vi "Write Credentials.vi"(8 "error in (no error)":errorcluster, 10 "Credentials":T1, 11 "AWS Core in":refnum<class "AWS Core.lvclass">) -> (0 "error out":errorcluster, 3 "AWS Core out":refnum<class "AWS Core.lvclass">)   [LabVIEW 2015, in "AWS Core.lvlib" / "AWS Core.lvclass"]
uses:
  AWS Core.lvclass
  AWS Credentials.ctl
  AWS Core.lvclass/AWS Core.ctl
  AWS Core.lvlib
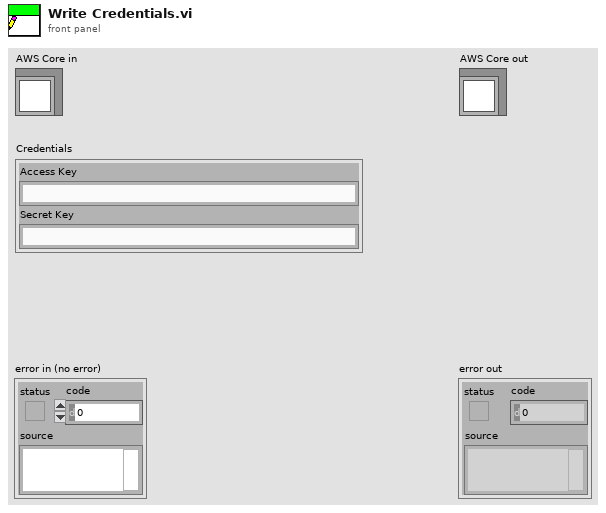
[diagram p1: front panel]
types:
  T1 = typedef "AWS Core.lvlib/AWS Credentials.ctl" = cluster{"Access Key":string, "Secret Key":string}
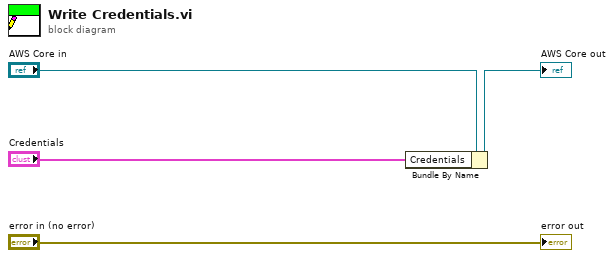
[diagram p0: block diagram]
diagram:
  n1 = Bundle By Name(cluster="AWS Core in", "Credentials"="Credentials") -> (→"AWS Core out":refnum<class "AWS Core.lvclass">)
  "error out" <- "error in (no error)"
